vi "unpackGates.vi"(2 "Current Waypoint":i16, 3 "Destinations Array":i64[][](array[numeric])=[[600, 500], [170, 290], [250, 950]]) -> (0 "Past Gate":i64[](array[numeric]), 1 "Current Gate":i64[](array[numeric]))   [LabVIEW 2012]
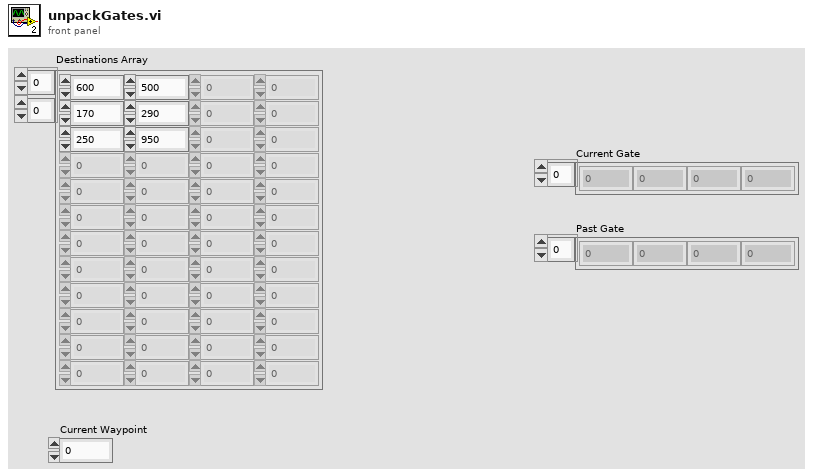
[diagram p1: front panel]
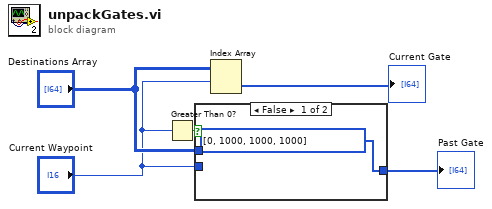
[diagram p0: block diagram]
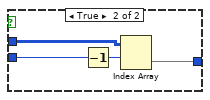
[diagram p2: hidden frame]
diagram:
  n1 = Greater Than 0?(x="Current Waypoint") -> (x > 0?=w2:bool)
  n2 = case shown="False" w2 {
    tunnel: "Destinations Array" -> [_ w10]
    tunnel: "Current Waypoint" -> [_ w8]
    tunnel: [i32[] [0, 1000, 1000, 1000] w7] -> w3
    frame False {
    }
    frame True {
      n3 = Decrement(x=w8) -> (x-1=w9:i16)
      n4 = Index Array(array=w10, index (row)=w9) -> (element=w7:i64[])  [unwired: 1 in]
    }
  }
  "Past Gate" <- w3
  n5 = Index Array(array="Destinations Array", index (row)="Current Waypoint") -> (element=→"Current Gate":i64[])  [unwired: 1 in]
